vi "REx - NART - Begin Point Calibration.vi"(1 "port number(3363)":u16=3363, 2 "machine name ()":string, 5 "Calibrate Config":T1={"Frequency, MHz"=2412, "TX Gain"=62, "Data Rate"="1,0,0", "Packet Length"=1000, "Packet Count"=2000000}, 11 "error in (no error)":errorcluster) -> (6 "Calibrate Config":T1={"Frequency, MHz"=2412, "TX Gain"=62, "Data Rate"="1,0,0", "Packet Length"=1000, "Packet Count"=2000000}, 15 "error out":errorcluster)   [LabVIEW 2011, in "ART2 Test Panel.lvlib" / "REx - NART - Begin Point Calibration.lvclass"]
uses:
  REx - NART - Begin Point Calibration.lvclass
  Components/ART2.llb/NART/Controls/Calibrate Config.ctl
  Components/ART2.llb/CART/Controls/Data Rates.ctl
  LVx Folder/LVx.lvclass
  ART2 Test Panel.lvlib
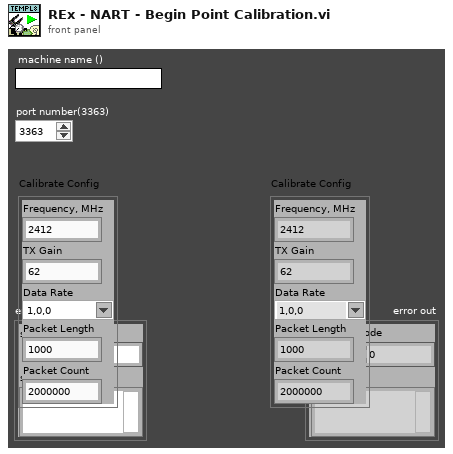
[diagram p1: front panel]
types:
  T1 = typedef "ART2 Test Panel.lvlib/Calibrate Config.ctl" = cluster{"Frequency, MHz":u32, "TX Gain":u32, "Data Rate":T2, "Packet Length":u32, "Packet Count":i32}
  T2 = typedef "ART2 Test Panel.lvlib/Data Rates.ctl" = string
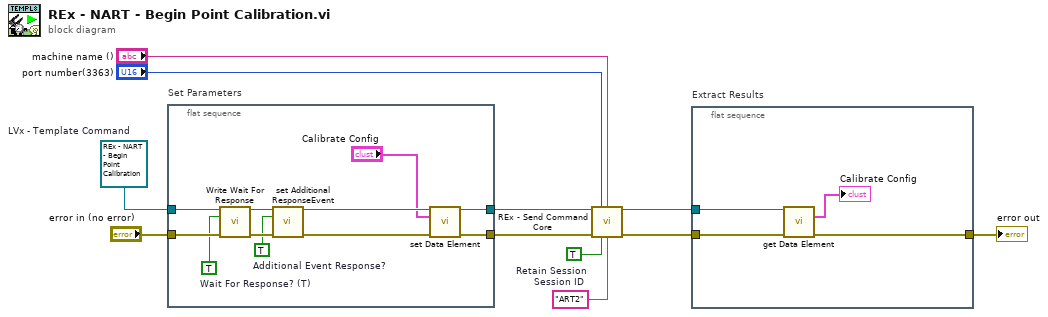
[diagram p0: block diagram]
diagram:
  w1 = "ART2"  # Session ID
  w3 = refnum<class "REx - NART - Begin Point Calibration.lvclass"> refnum  # LVx - Template Command
  w4 = TRUE  # Retain Session
  n1 = flat-sequence "Set Parameters" {
    tunnel: [w13] -> w11
    tunnel: "error in (no error)" -> [w19]
    tunnel: [w15] -> w8
    tunnel: w3 -> [w20]
    frame #0 {
      w17 = TRUE  # Additional Event Response?
      w18 = TRUE  # Wait For Response? (T)
      n2 = call "Write Wait For Response.vi"("LVx.lvclass in"=w20, "Wait For Response? (T)"=w18, "error in (no error)"=w19) -> ("LVx.lvclass out"=w21:refnum<class "REx - NART - Begin Point Calibration.lvclass">, "error out"=w22:errorcluster)  [unwired: 11 in]
      n3 = call "set Additional ResponseEvent.vi"("LVx in"=w21, "Fire Additional Event for Response?"=w17, "error in (no error)"=w22) -> ("LVx out"=w14:refnum<class "REx - NART - Begin Point Calibration.lvclass">, "error out"=w16:errorcluster)  [unwired: 11 in]
      n4 = call "set Data Element.vi"("LVx - Template Command in"=w14, "Calibrate Config"="Calibrate Config", "error in (no error)"=w16) -> ("LVx - Template Command out"=w13:refnum<class "REx - NART - Begin Point Calibration.lvclass">, "error out"=w15:errorcluster)  [unwired: 11 in]
    }
  }
  n5 = call "REx - Send Command Core.vi"("LVx Command in"=w11, "port number(3363)"="port number(3363)", "machine name (LocalApp:\"\")"="machine name ()", "error in (no error)"=w8, "Retain Session (F)"=w4, "Session ID"=w1) -> ("LVx Command response"=w5:refnum<class "REx - NART - Begin Point Calibration.lvclass">, "error out"=w10:errorcluster)  [unwired: 8 in]
  n6 = flat-sequence "Extract Results" {
    tunnel: w10 -> [w24]
    tunnel: w5 -> [w26]
    tunnel: [w23] -> w2
    frame #0 {
      n7 = call "get Data Element.vi"("LVx - Template Command in"=w26, "error in (no error)"=w24) -> ("Calibrate Config"=→"Calibrate Config":T1, "error out"=w23:errorcluster)  [unwired: 11 in, 1 out]
    }
  }
  "error out" <- w2
